vi "CoriFlowBFS1Plus_Init.vi"(0 "object in":refnum<class "CoriFlowBFS1Plus.lvclass">, 2 "VISA resource name":refnum<visa-resource-name>, 3 "Filter(0-1)Min-Max":dbl min=0.0 max=1.0, 4 "SW Buffer Size":i32, 5 "error in (no error)":errorcluster) -> (14 "object out":refnum<class "CoriFlowBFS1Plus.lvclass">, 19 "error out":errorcluster)   [LabVIEW 2021, in "CoriFlowBFS1Plus.lvclass"]
uses:
  CoriFlowBFS1Plus.lvclass
  CoriFlowBFS1Plus.lvclass/CoriFlowBFS1Plus.ctl
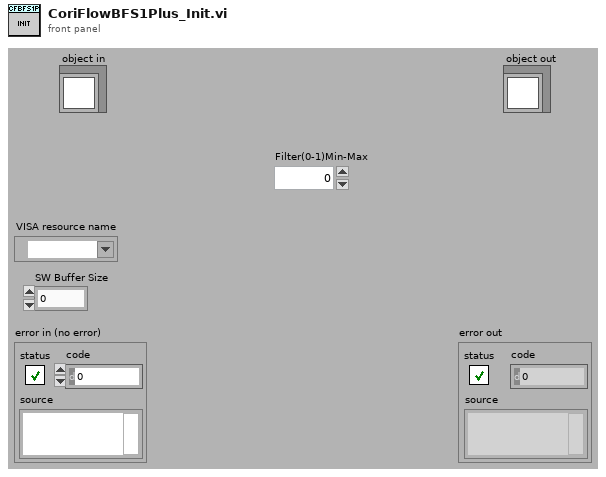
[diagram p1: front panel]
types:
  T1 = cluster{"Message":string, "Message Data":variant}
  T2 = cluster{"Cluster":cluster{"Density_g_L":sgl, "FLow(ul/min)":sgl, "Temperature(C)":sgl}, "current time":timestamp}
  T3 = typedef "Z_BFS_type.ctl" = cluster{"VISA_Name":refnum<visa-resource-name>, "density_g_L":dbl, "Capacity":dbl, "Capacity units conversion":dbl}
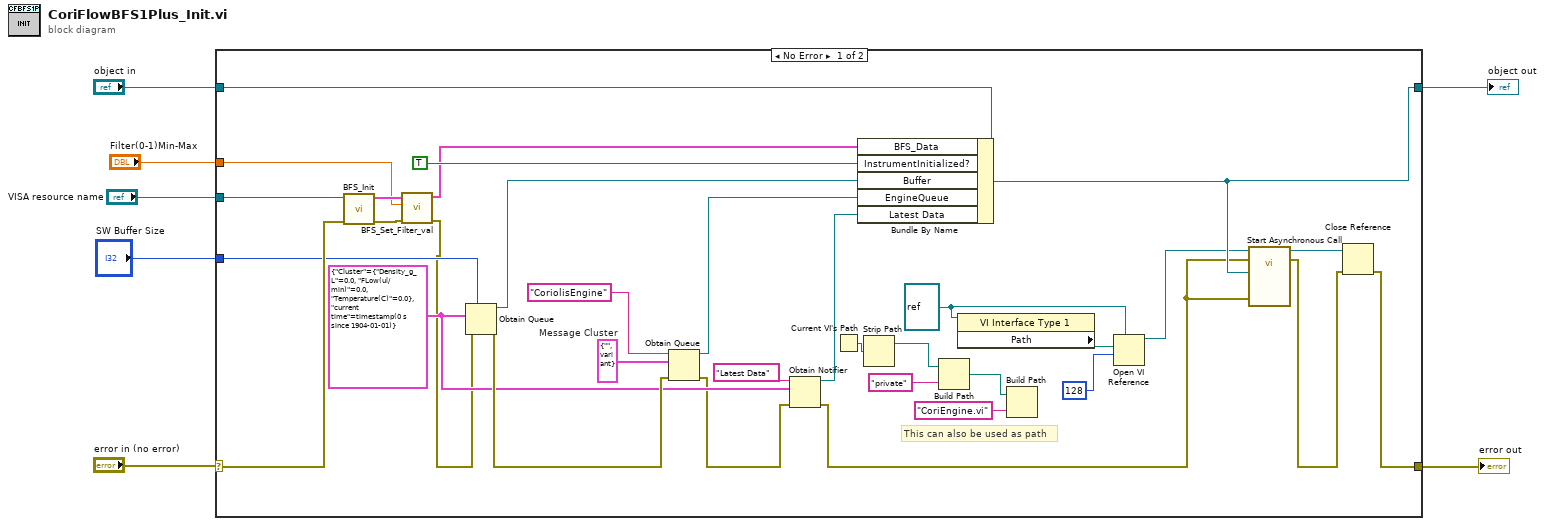
[diagram p0: block diagram]
diagram:
  n1 = case shown="No Error" "error in (no error)" {
    selector: "error in (no error)" -> [w38 w41]
    tunnel: "object in" -> [w40 w42]
    tunnel: [w15 w42] -> w6
    tunnel: [w10 w41] -> w4
    tunnel: "VISA resource name" -> [w39 _]
    tunnel: "Filter(0-1)Min-Max" -> [w34 _]
    tunnel: "SW Buffer Size" -> [w33 _]
    frame No Error {
      w9 = refnum<vi> refnum ("type specifier VI Refnum (for type only)")
      w31 = T1 {"Message"="", "Message Data"=variant}  # Message Cluster
      w27 = T2 {"Cluster"={"Density_g_L"=0.0, "FLow(ul/min)"=0.0, "Temperature(C)"=0.0}, "current time"=timestamp(0 s since 1904-01-01)}
      # "This can also be used as path"
      n2 = call "BFS_Init.vi"("error in"=w38, "VISA resource name"=w39) -> ("error out"=w23:errorcluster, "BFS_Out"=w36:T3)  [unwired: 8 in]
      n3 = call "BFS_Set_Filter_val.vi"("error in (no error)"=w23, "Sensor_Filter_0_to_1"=w34, "BFS_type_In"=w36) -> ("error out"=w22:errorcluster, "BFS_type_Out"=w35:T3)  [unwired: 7 in]
      n4 = Obtain Queue(max queue size (-1, unlimited)=w33, element data type=w27, error in (no error)=w22) -> (queue out=w32:refnum<queue>, error out=w30:errorcluster)  [unwired: 2 in, 1 out]
      n5 = Obtain Queue(name (unnamed)="CoriolisEngine", element data type=w31, error in (no error)=w30) -> (queue out=w28:refnum<queue>, error out=w25:errorcluster)  [unwired: 2 in, 1 out]
      n6 = Obtain Notifier(name (unnamed)="Latest Data", notification data type=w27, error in (no error)=w25) -> (notifier out=w24:refnum<notifier>, error out=w14:errorcluster)  [unwired: 1 in, 1 out]
      n7 = Current VI's Path() -> (path=w19:path)
      n8 = Bundle By Name(cluster=w40, "BFS_Data"=w35, "InstrumentInitialized?"=TRUE, "Buffer"=w32, "EngineQueue"=w28, "Latest Data"=w24) -> (w15:refnum<class "CoriFlowBFS1Plus.lvclass">)
      n9 = Strip Path(path=w19) -> (stripped path=w20:path)  [unwired: 1 out]
      n10 = Build Path(base path=w20, name or relative path="private") -> (appended path=w21:path)
      n11 = property class="VI Interface Type 1"(reference=w9) -> ("Path"=w8:path)  [unwired: 1 in, 2 out]
      n12 = Build Path(base path=w21, name or relative path="CoriEngine.vi") -> ()  [unwired: 1 out]
      n13 = Open VI Reference(type specifier VI Refnum (for type only)=w9, vi path=w8, options=128) -> (vi reference=w13:refnum<vi>)  [unwired: 3 in, 1 out]
      n14 = call-by-ref "Start Asynchronous Call"(reference=w13, error in=w14, "object in"=w15, 5:"error in (no error)"=w14) -> (reference out=w12:refnum<vi>, error out=w11:errorcluster)  [unwired: 16 in, 2 out]
      n15 = Close Reference(reference=w12, error in (no error)=w11) -> (error out=w10:errorcluster)
    }
    frame Error {
    }
  }
  "object out" <- w6
  "error out" <- w4
